vi "Zip_a_Folder.vi"(8 "error in (no error)":errorcluster, 9 "DestinationPathFolder":path, 10 "Zipping....":refnum<vi>, 11 "object in":refnum<class "Crypter.lvclass">) -> (0 "error out":errorcluster, 3 "object out":refnum<class "Crypter.lvclass">)   [LabVIEW 2016, in "Crypter.lvclass"]
uses:
  Crypter.lvclass
  Crypter.lvclass/Crypter.ctl
  <userlib>/_OpenG.lib/file/file.llb/Strip Path Extension - Path__ogtk.vi
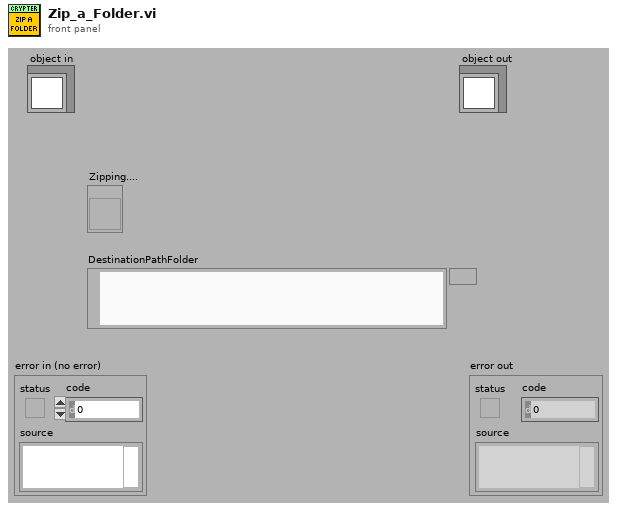
[diagram p1: front panel]
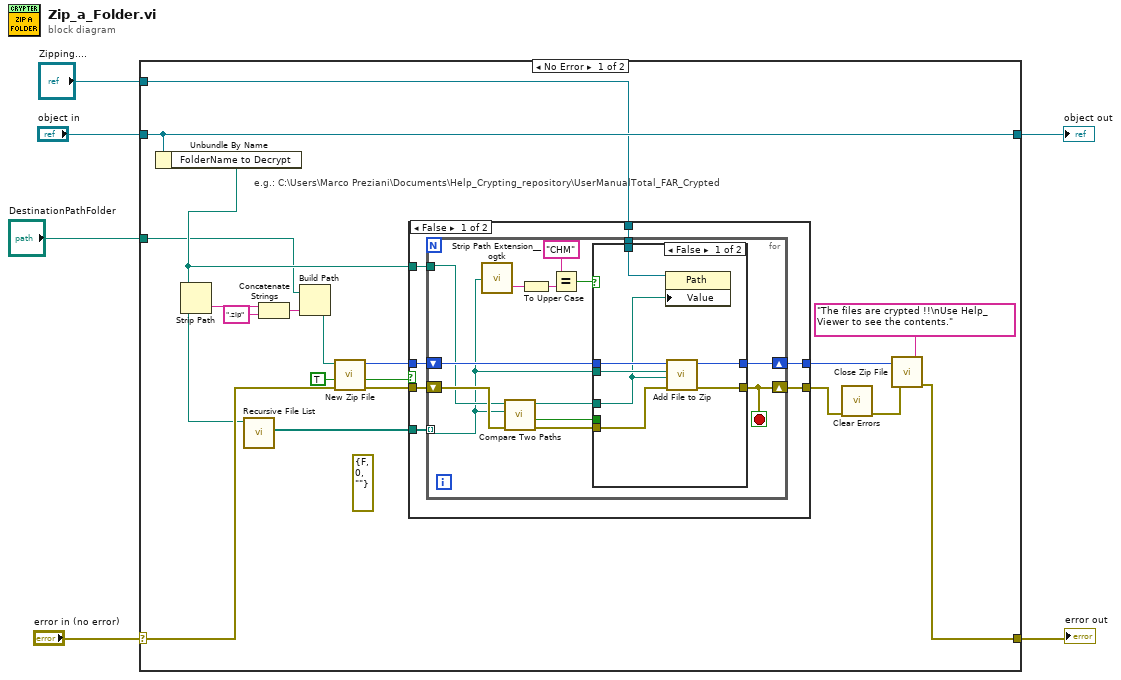
[diagram p0: block diagram]
diagram:
  n1 = case shown="No Error" "error in (no error)" {
    selector: "error in (no error)" -> [w21 w59]
    tunnel: [w13 w59] -> w5
    tunnel: [w25 w58] -> w3
    tunnel: "object in" -> [w25 w58]
    tunnel: "Zipping...." -> [w8 _]
    tunnel: "DestinationPathFolder" -> [w7 _]
    frame No Error {
      (unwired) errorcluster {"status"=FALSE, "code"=0, "source"=""} ("error out")
      # "e.g.: C:\\Users\\Marco Preziani\\Documents\\Help_Crypting_repository\\UserManualTotal_FAR_Crypted"
      n2 = Unbundle By Name(w25) -> ("FolderName to Decrypt"=w10:path)
      n3 = Strip Path(path=w10) -> (name=w20:string)  [unwired: 1 out]
      n4 = call <vilib>:"Recursive File List.vi"("Folder Path"=w10) -> ("All Files in Dir"=w16:path[])  [unwired: 6 in, 4 out]
      n5 = Concatenate Strings(w20, ".zip" ("element")) -> (w18:string)
      n6 = Build Path(base path=w7, name or relative path=w18) -> (appended path=w17:path)
      n7 = call <vilib>:"New Zip File.vi"("error in (no error)"=w21, "confirm overwrite? (F)"=TRUE, "target"=w17) -> ("error out"=w9:errorcluster, "cancelled"=w23:bool, "zip file out"=w24:i64)  [unwired: 2 in]
      n8 = case shown="False" w23 {
        tunnel: w9 -> [w32 w57]
        tunnel: w24 -> [w31 w56]
        tunnel: [w27 w57] -> w12
        tunnel: w16 -> [w29 _]
        tunnel: w10 -> [w30 _]
        tunnel: [w28 w56] -> w14
        tunnel: w8 -> [w26 _]
        frame False {
          n9 = for {
            shift-right: [w41] -> w27
            shift-left: w32 -> [w45]
            tunnel: w30 -> [w39]
            tunnel: w29 -> [w38] mode=indexing
            shift-right: [w44] -> w28
            shift-left: w31 -> [w46]
            tunnel: w26 -> [w33]
            stop <- w41 stop-if-true
            n10 = call-poly <userlib>:"Strip Path Extension__ogtk.vi"("path"=w38) -> ("extension"=w37:string)  [unwired: 1 out]
            n11 = call <vilib>:"Compare Two Paths.vi"("error in (no error)"=w45, "Path 2"=w38, "Path 1"=w39) -> ("error out"=w42:errorcluster, "Path 2 Relative to Path 1?"=w40:bool, "Relative Path from 1 to 2"=w43:path)  [unwired: 5 in, 1 out]
            n12 = To Upper Case(1:w37) -> (0:w35:string)
            n13 = Equal?(x="CHM", y=w35) -> (x = y?=w34:bool)
            n14 = case shown="False" w34 {
              tunnel: w46 -> [w53 w55]
              tunnel: [w52 w55] -> w44
              tunnel: w43 -> [w47 _]
              tunnel: w42 -> [w51 w54]
              tunnel: [w50 w54] -> w41
              tunnel: w40 -> [_ _]
              tunnel: w38 -> [w49 _]
              tunnel: w33 -> [w48 _]
              frame False {
                n15 = property class="Path"(reference=w48, "Value"=w47) -> ()  [unwired: 1 in, 2 out]
                n16 = call <vilib>:"Add File to Zip.vi"("error in (no error)"=w51, "destination path in zip"=w47, "source file path"=w49, "zip file in"=w53) -> ("error out"=w50:errorcluster, "zip file out"=w52:i64)  [unwired: 6 in]
              }
              frame True {
              }
            }
          }
        }
        frame True {
        }
      }
      n17 = call <vilib>:"Clear Errors.vi"("error in (no error)"=w12) -> ("error out"=w11:errorcluster)  [unwired: 5 in, 1 out]
      n18 = call <vilib>:"Close Zip File.vi"("error in (no error)"=w11, "comments"="The files are crypted !!\nUse Help_Viewer to see the contents.", "zip file in"=w14) -> ("error out"=w13:errorcluster)  [unwired: 4 in]
    }
    frame Error {
    }
  }
  "error out" <- w5
  "object out" <- w3
